vi "2D Matrix (Normal).vi"(10 "nRows":i32=1, 11 "nCols":i32=1) -> (3 "Normal Matrix":T1 format="%_8f")   [LabVIEW 2014]
uses:
  <vilib>/Analysis/Matrix/Datatypes/RealMatrix.ctl
  <vilib>/gmath/statdist.llb/Normal Random.vi
  <vilib>/gmath/NI_Gmath.lvlib
  <vilib>/Analysis/Matrix/NI_Matrix.lvlib
panel:
  in  "std":dbl=1.0 format="%#_13g"
  in  "mean":dbl format="%#_13g"
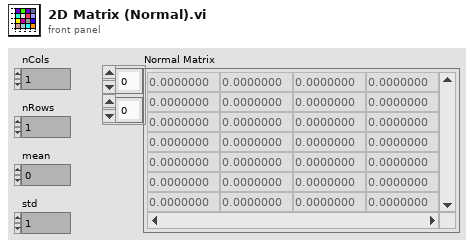
[diagram p1: front panel]
types:
  T1 = typedef "NI_Matrix.lvlib/RealMatrix.ctl" = dbl[][]
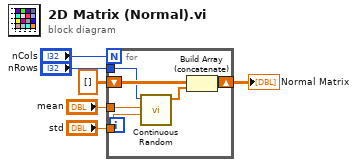
[diagram p0: block diagram]
diagram:
  n1 = for {
    N: "nCols" -> [_]
    tunnel: "std" -> [w12]
    tunnel: "mean" -> [w11]
    shift-right: [w9] -> w4
    shift-left: T1 [] ("Real Matrix") -> [w8]
    tunnel: "nRows" -> [w7]
    n2 = call-poly <vilib>:"Continuous Random.vi"("std"=w12, "mean"=w11, "samples"=w7) -> ("normal random data"=w10:dbl[])  [unwired: 7 in, 1 out]
    n3 = Build Array (concatenate)(w8, w10) -> (w9:T1)
  }
  "Normal Matrix" <- w4
